vi "Demo_1.vi"() -> ()   [LabVIEW 2020]
panel:
  in  "y":dbl
  out "Tank":dbl(slide) scale=0.0..10.0
  in  "Dial":dbl(knob) scale=0.0..100.0
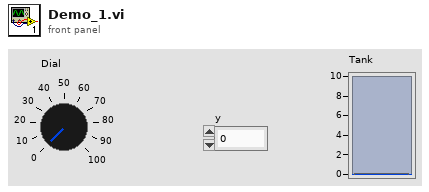
[diagram p1: front panel]
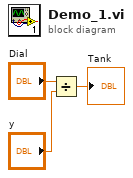
[diagram p0: block diagram]
diagram:
  n1 = Divide(x="Dial", y="y") -> (x/y=→"Tank":dbl)
